vi "DMC1000B_1 OutBit.vi"(8 "error in (no error)":errorcluster, 10 "BL":bool, 11 "IO_Output_1 Select":T1=enum."M_OUT22") -> (0 "error out":errorcluster)   [LabVIEW 2019]
uses:
  Ctrl/DMC1000B_1 SelectOutput.ctl
  IO_Class/IOCard.lvclass
panel:
  in  "CardIndex":i32
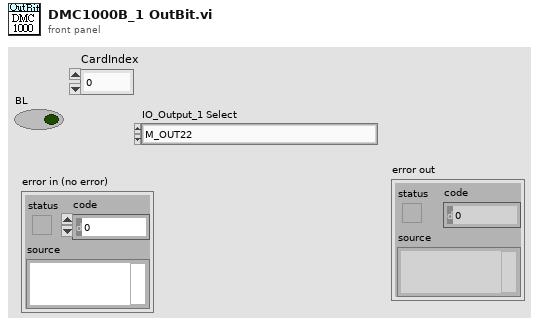
[diagram p1: front panel]
types:
  T1 = typedef "DMC1000B_1 SelectOutput.ctl" = enum16{"M_Out0預備", "M_OUT01蜂鳴器", "M_OUT02紅燈", "M_OUT03綠燈", "M_OUT04黃燈", "M_OUT05上頂固定位氣缸電磁閥", "M_OUT06到料阻擋氣缸電磁閥", "M_OUT07向前機台發出要料#1信號", "M_OUT08向前機台發出要料#2信號", "M_OUT09向後機台發出有料#3信號", "M_OUT10向後機台發出有料#4信號", "M_OUT11接駁台馬達啟動開/關", "M_OUT12接駁台馬達慢速", "M_OUT13抽風機開/關", "M_OUT14上視覺上光源", "M_OUT15DC吹風扇開/關", "M_OUT16Z軸煞車釋放", "M_OUT17", "M_OUT18", "M_OUT19", "M_OUT20", "M_OUT21", "M_OUT22", "M_OUT23", "M_OUT24", "M_OUT25第一軸SEVON1伺服使能信號", "M_OUT26第二軸SEVON2伺服使能信號", "M_OUT27第三軸SEVON3伺服使能信號"}
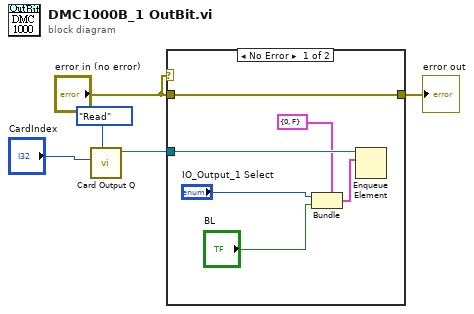
[diagram p0: block diagram]
diagram:
  n1 = call "Card Output Q.vi"("Action"=enum16{"Initial", "Write", "Read", "Release"}."Read", "CardIndex"="CardIndex") -> ("Output Q Out"=w1:refnum<queue>)  [unwired: 8 in, 1 out]
  n2 = case shown="No Error" "error in (no error)" {
    tunnel: "error in (no error)" -> [w10 w12]
    tunnel: [w10 w12] -> w5
    tunnel: w1 -> [w11 _]
    frame No Error {
      n3 = Bundle(cluster=cluster{"Index":i32, "BL":bool} {"Index"=0, "BL"=FALSE} ("element"), "Index"="IO_Output_1 Select", "BL"="BL") -> (w6:cluster{"Index":i32, "BL":bool})
      n4 = Enqueue Element(queue=w11, element=w6) -> ()  [unwired: 2 in, 3 out]
    }
    frame Error {
    }
  }
  "error out" <- w5
